vi "Live window-Image display select.vi"(10 "Which image display?":T1) -> (2 "Image display ref":T2)   [LabVIEW 2020]
uses:
  Typedefs/Image display ref.ctl
  Typedefs/Left-Right enum.ctl
  Globals/gl_Windows Ctrl refs.vi
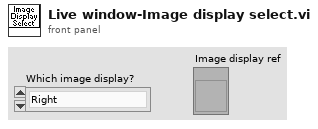
[diagram p1: front panel]
types:
  T1 = typedef "Left-Right enum.ctl" = enum16{"Right", "Left"}
  T2 = typedef "Image display ref.ctl" = refnum<vi>
  T3 = typedef "Live window-ctrl refs.ctl" = cluster{"This VI":refnum<vi>, "Pane":refnum<vi>, "Show REF Image Left":refnum<vi>, "Show REF Image Right":refnum<vi>, "Snapshot":refnum<vi>, "Left Image Palette":refnum<vi>, "Right Image Palette":refnum<vi>, "Left Channel":refnum<vi>, "Right Channel":refnum<vi>, "Left image intensity":refnum<vi>, "Right image intensity":refnum<vi>, "Left Image Display":T2, "Right Image Display":T2, "Refresh rate ind (Hz)":refnum<vi>, "Acq rate ind (Hz)":refnum<vi>, "Stop (ind)":refnum<vi>}
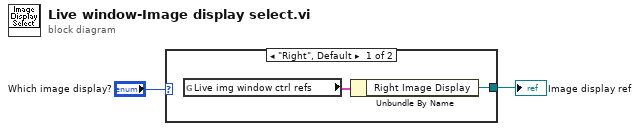
[diagram p0: block diagram]
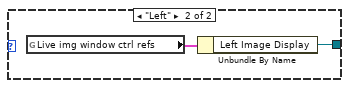
[diagram p2: hidden frame]
diagram:
  n1 = case shown="\"Right\", Default" "Which image display?" {
    tunnel: [w3 w5] -> w2
    frame "Right", Default {
      n2 = global read "gl_Windows Ctrl refs.vi" "Live img window ctrl refs"() -> (w4:T3)
      n3 = Unbundle By Name(w4) -> ("Right Image Display"=w3:T2)
    }
    frame "Left" {
      n4 = global read "gl_Windows Ctrl refs.vi" "Live img window ctrl refs"() -> (w6:T3)
      n5 = Unbundle By Name(w6) -> ("Left Image Display"=w5:T2)
    }
  }
  "Image display ref" <- w2
